vi "RT Loop - Interlock and Post Mortem Data.vi"(8 "error in (no error)":errorcluster, 9 "Master Configuration":T1, 10 "FPGA Subsystem":refnum<queue>, 11 "Message Handler":refnum<queue>) -> ()   [LabVIEW 2014]
uses:
  support/Message Queue/Message Cluster.ctl
  controls/Master Configuration.ctl
  controls/EPICS Configuration.ctl
  controls/FPGA VI Reference.ctl
  <vilib>/Platform/TimedLoop/XDataNode/timing_clust.ctl
  <vilib>/Platform/TimedLoop/XDataNode/nitl_modes.ctl
  <vilib>/Platform/TimedLoop/XDataNode/wakeup.ctl
  Globals/Global - Monitoring Variables.vi
  <vilib>/rvi/errors/niLvFpgaAdjustHostInterfaceError.vi
  Globals/Global - Configuration Options.vi
  <vilib>/Platform/TimedLoop/XDataNode/XDataNode.xnode
  <vilib>/rvi/interface/nirviReadWriteControl/nirviReadWriteControl.xnode
  <vilib>/rvi/interface/nirviMethod/nirviMethod.xnode
  support/Message Queue/Message Queue.lvlib
  <vilib>/FPGAPlugInAG/Dynamic/niLvFpga_ReadFifo_Dynamic.vi
  <vilib>/rvi/errors/niLvFpgaMergeErrorWithErrorCode.vi
  <vilib>/Platform/TimedLoop/XDataNode/XDNodeRunTimeDep.lvlib
  <vilib>/rvi/interface/Simulation/niFpgaSimulationCallBeginRW.vi
  NiFpgaLv.dll
  <vilib>/FPGAPlugInAG/Dynamic/niLvFpga_StopFifo_Dynamic.vi
panel:
  in  "stop":bool
  out "Finished Late?":bool
  out "Iteration Duration":i64
  out "error out 2":errorcluster
  out "error out":errorcluster
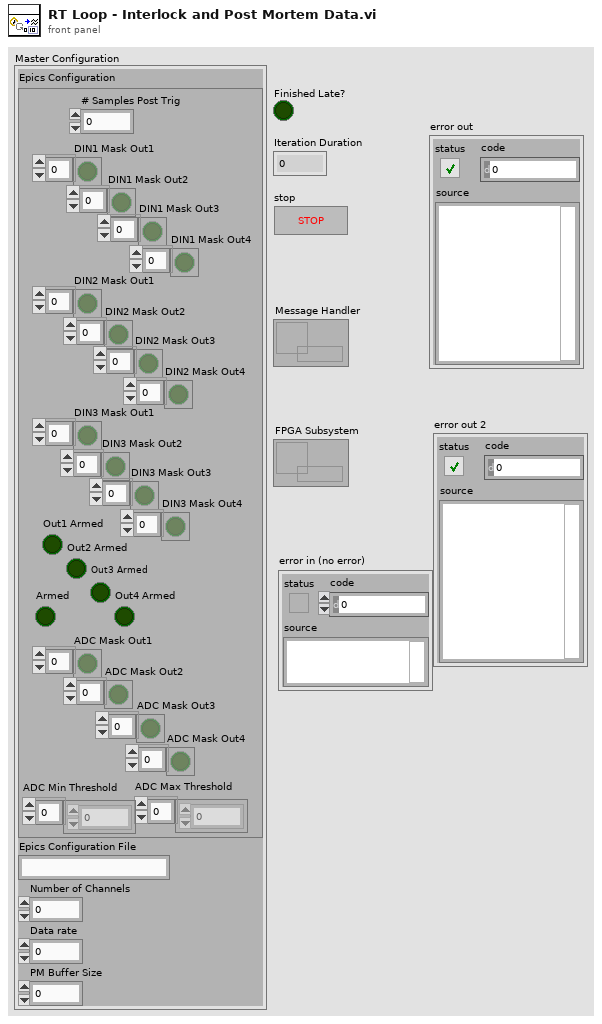
[diagram p1: front panel]
types:
  T1 = typedef "Master Configuration.ctl" = cluster{"Epics Configuration":T2, "Epics Configuration File":string, "Number of Channels":u8, "Data rate":u32, "PM Buffer Size":u32}
  T2 = typedef "EPICS Configuration.ctl" = cluster{"DIN1 Mask Out1":bool[], "# Samples Post Trig":u32, "Armed":bool, "ADC Mask Out1":bool[], "ADC Max Threshold":dbl[], "ADC Min Threshold":dbl[], "DIN1 Mask Out2":bool[], "DIN1 Mask Out3":bool[], "DIN1 Mask Out4":bool[], "Out3 Armed":bool, "Out1 Armed":bool, "Out4 Armed":bool, "Out2 Armed":bool, "DIN2 Mask Out1":bool[], "DIN2 Mask Out2":bool[], "DIN2 Mask Out3":bool[], "DIN2 Mask Out4":bool[], "DIN3 Mask Out1":bool[], "DIN3 Mask Out2":bool[], "DIN3 Mask Out3":bool[], "DIN3 Mask Out4":bool[], "ADC Mask Out2":bool[], "ADC Mask Out3":bool[], "ADC Mask Out4":bool[]}
  T3 = typedef "FPGA VI Reference.ctl" = refnum<k20>
  T4 = typedef "XDNodeRunTimeDep.lvlib/timing_clust.ctl" = cluster{"Expected End [f-1]":u64, "Actual End [f-1]":u64, "Finished Late? [f-1]":bool, "Expected End [i-1]":u64, "Actual End [i-1]":u64, "Finished Late? [i-1]":bool, "Expected Start [i]":u64, "Actual Start [i]":u64, "Expected Start [f]":u64, "Actual Start [f]":u64, "Source Name":string, "Structure Name":string, "Period":i64, "Deadline":i64, "Offset":i64, "Start":i64, "Priority":i32, "Timeout":i32, "Mode":T5, "Wakeup Reason":T6, "Error":errorcluster, "Source Type":string, "Secondary Source Type":string, "Global End Time":u64, "Global Start Time":u64, "Frame Duration":u64, "Iteration Duration":u64, "Assigned CPU":i32, "I/O Scan Engine Mode":u32}
  T5 = typedef "XDNodeRunTimeDep.lvlib/nitl_modes.ctl" = enum32{"No Change", "Process missed periods, maintain original phase", "Discard missed periods, maintain original phase", "Process missed periods, ignore original phase", "Discard missed periods, ignore original phase"}
  T6 = typedef "XDNodeRunTimeDep.lvlib/wakeup.ctl" = enum32{"Normal", "Aborted", "Asynchronous wakeup", "Timing source error", "Timed loop error", "Timeout"}
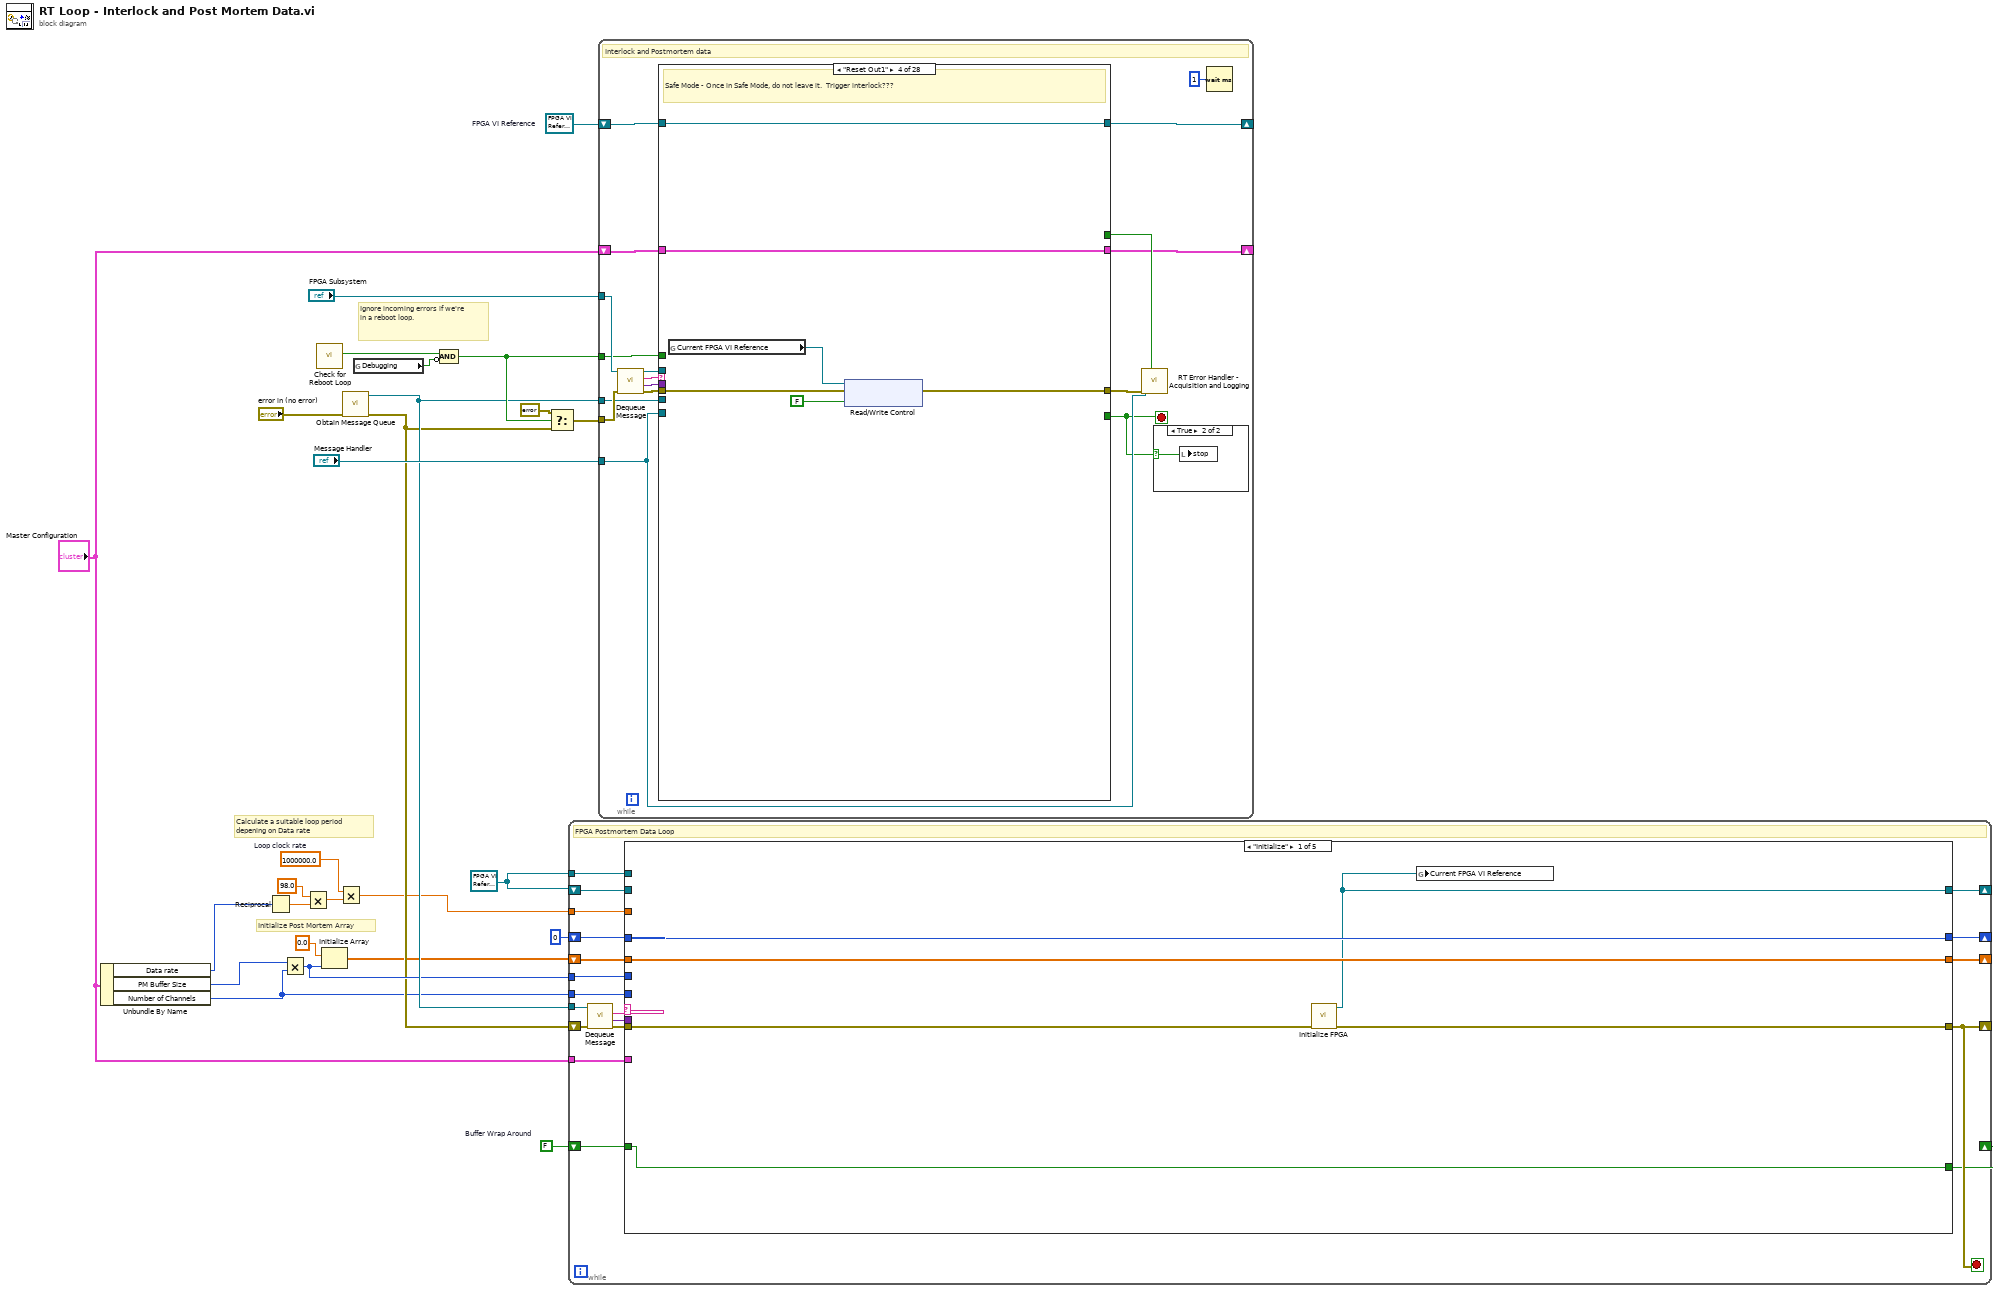
[diagram p0: block diagram]
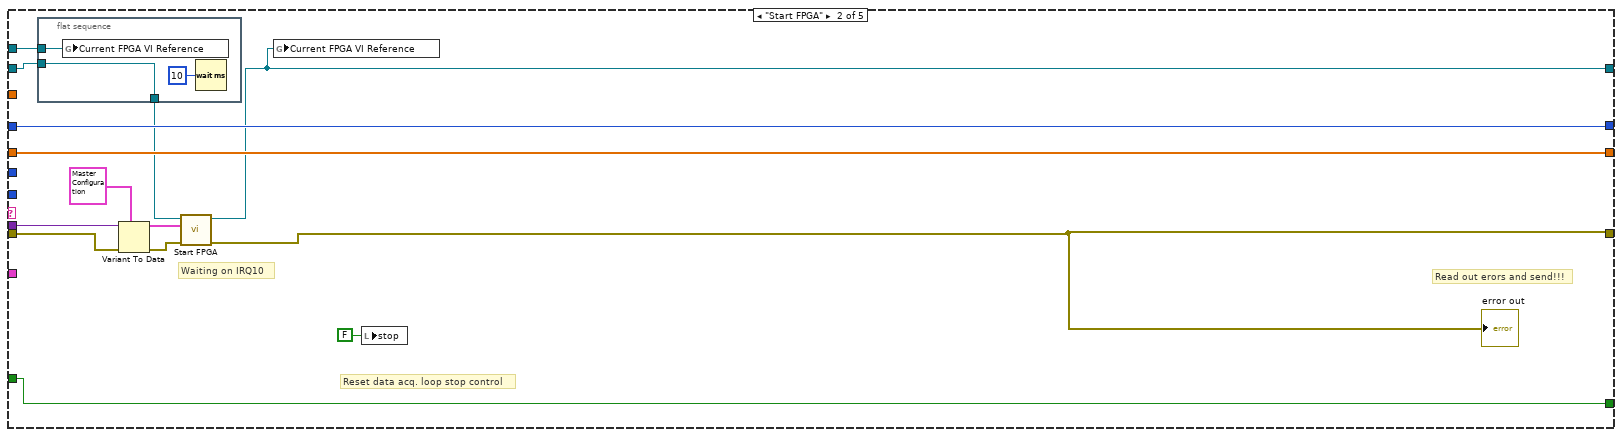
[diagram p2: hidden frame]
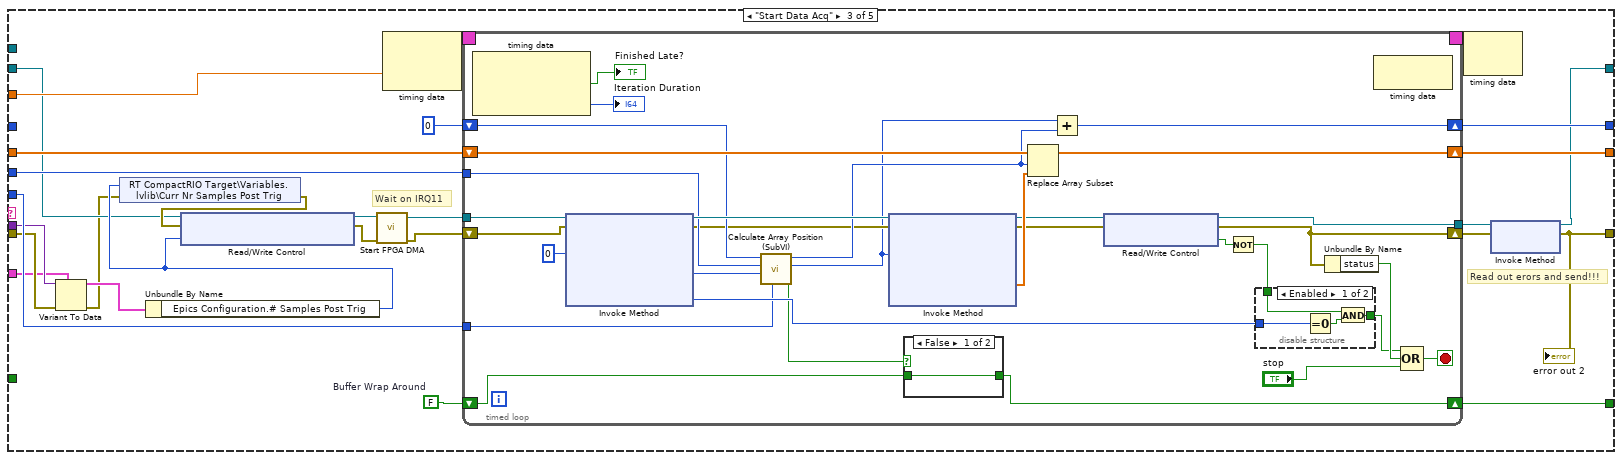
[diagram p3: hidden frame]
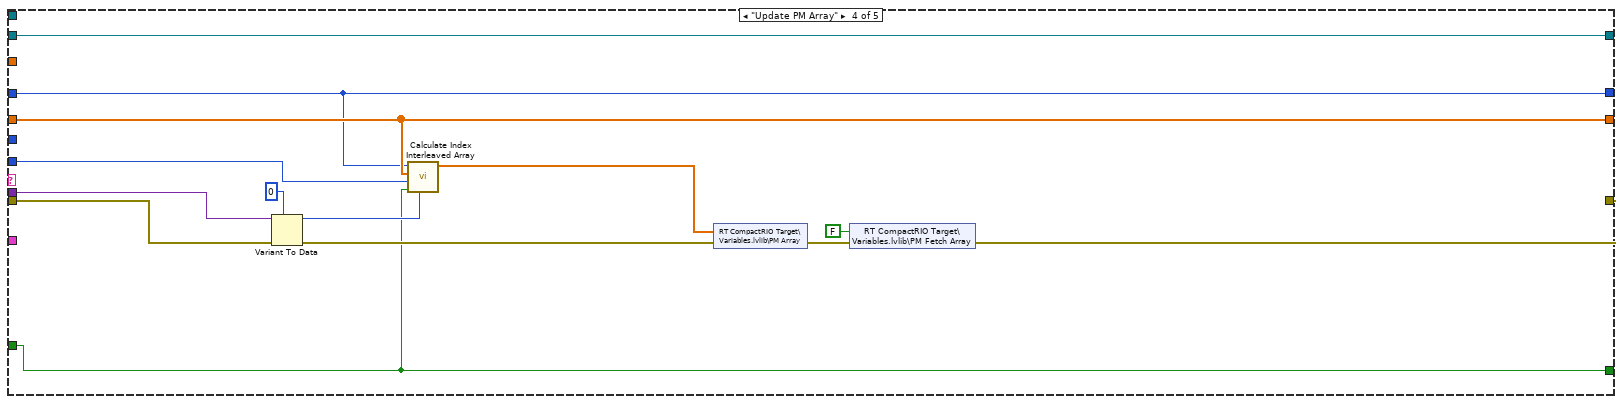
[diagram p6: hidden frame]
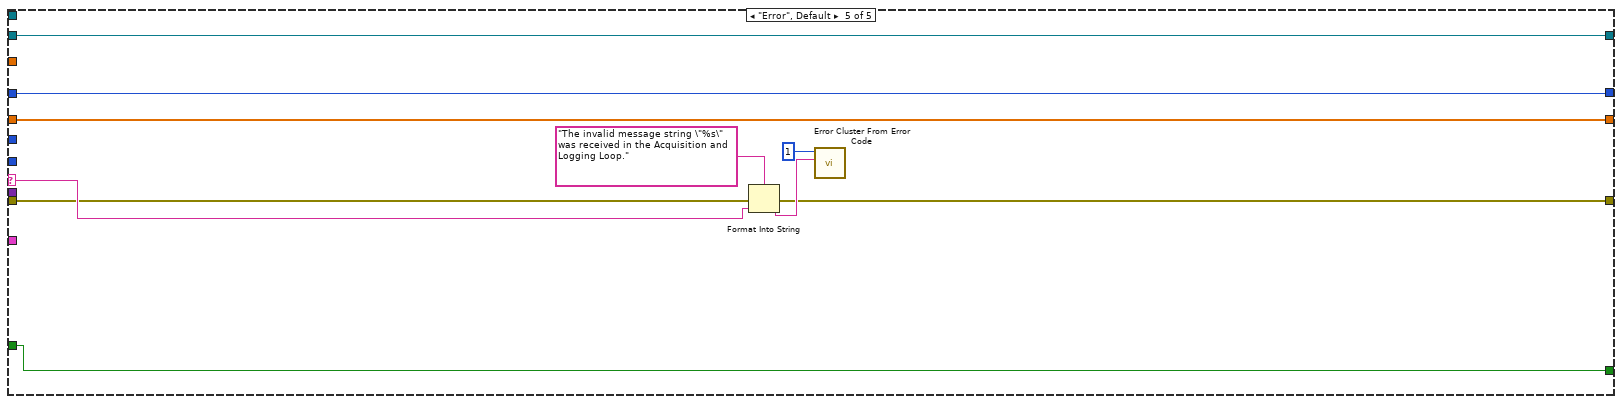
[diagram p7: hidden frame]
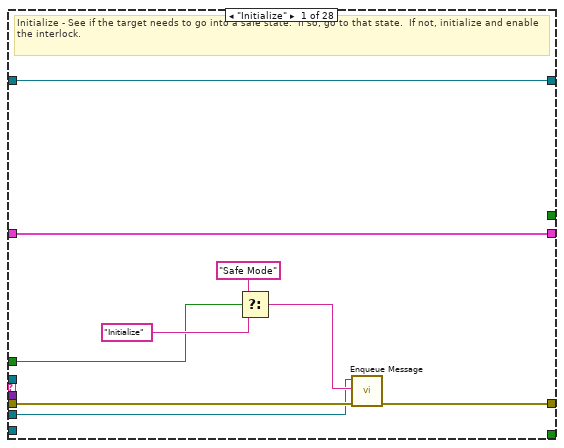
[diagram p9: hidden frame]
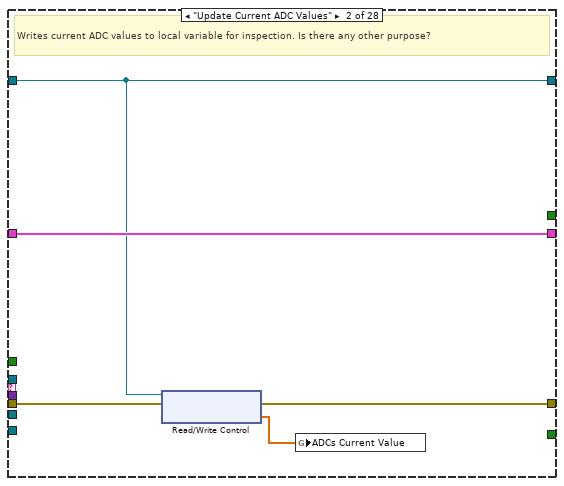
[diagram p10: hidden frame]
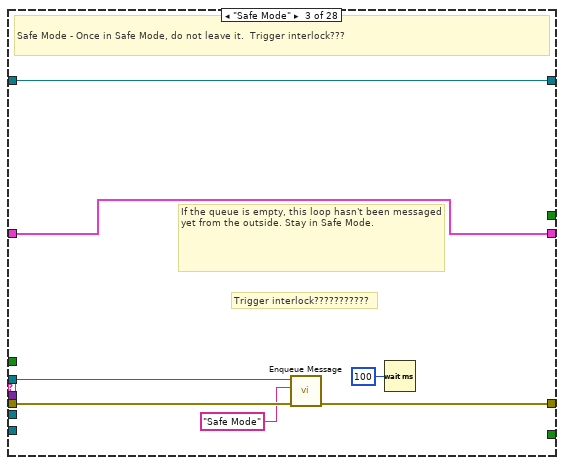
[diagram p11: hidden frame]
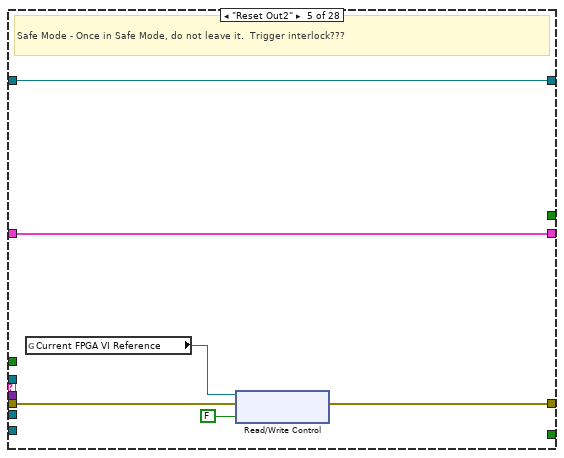
[diagram p12: hidden frame]
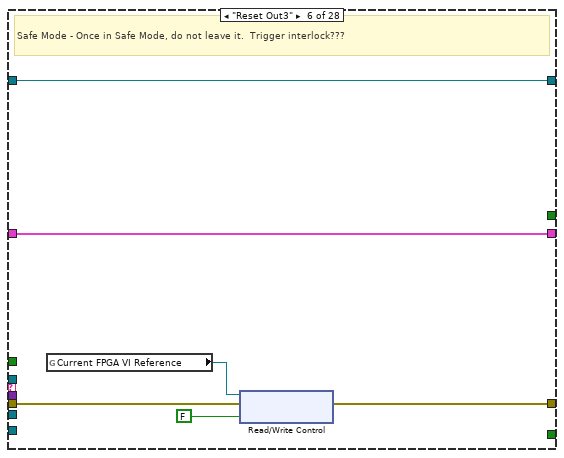
[diagram p13: hidden frame]
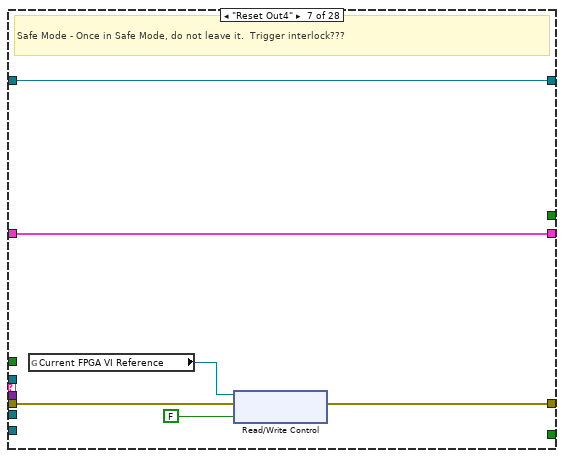
[diagram p14: hidden frame]
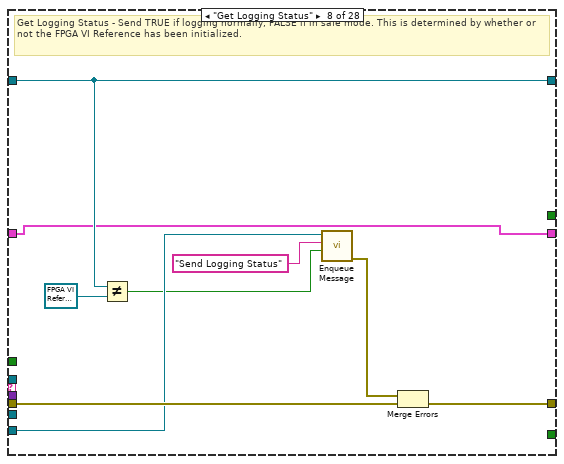
[diagram p15: hidden frame]
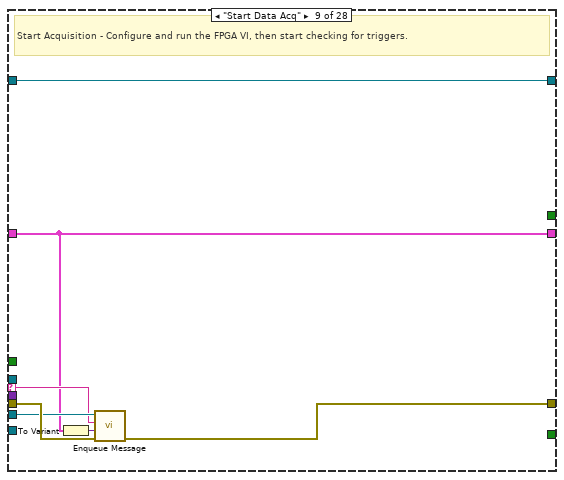
[diagram p16: hidden frame]
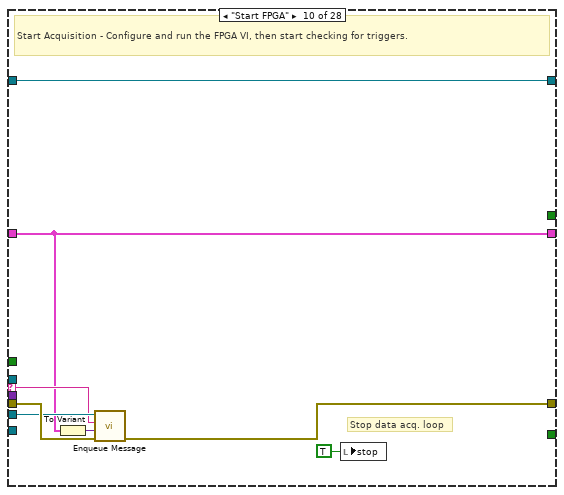
[diagram p17: hidden frame]
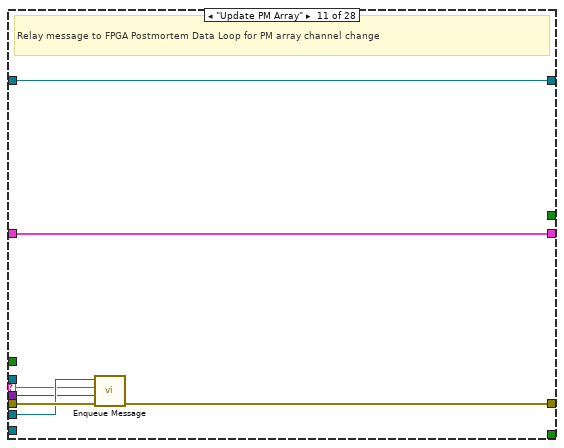
[diagram p18: hidden frame]
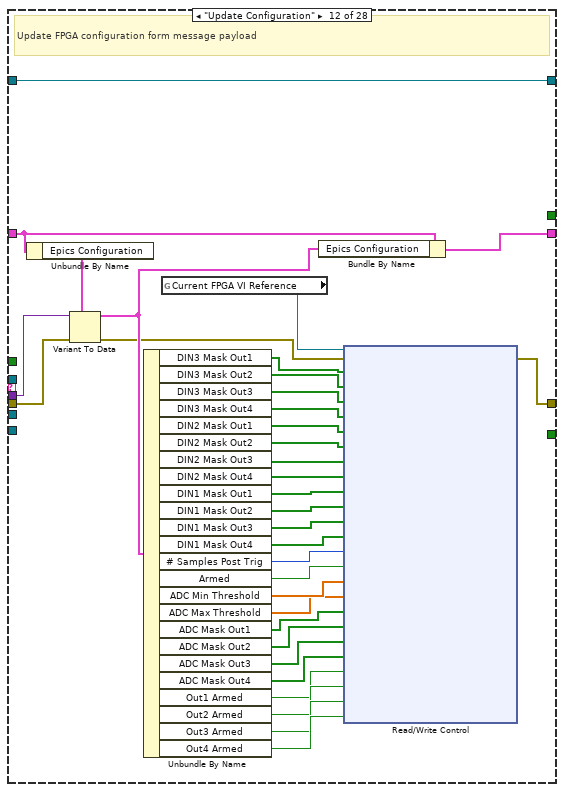
[diagram p19: hidden frame]
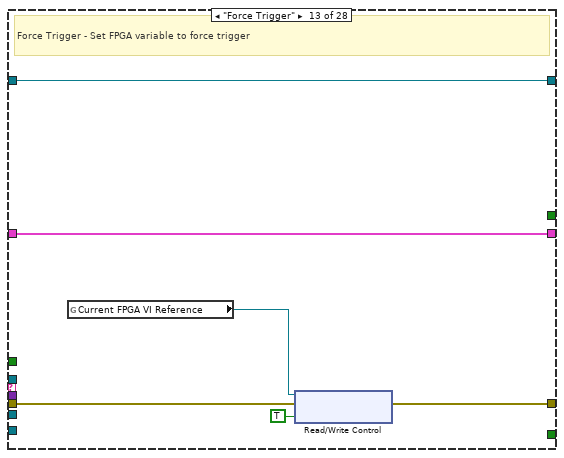
[diagram p20: hidden frame]
diagram:
  w1 = FALSE  # Buffer Wrap Around
  w4 = 1000000.0  # Loop clock rate
  w10 = T3 refnum ("FPGA VI Reference")
  w24 = T3 refnum  # FPGA VI Reference
  # "Calculate a suitable loop period\ndepening on Data rate"
  # "Initialize Post Mortem Array"
  # "Ignore incoming errors if we're in a reboot loop."
  n1 = Unbundle By Name("Master Configuration") -> ("Data rate"=w8:u32, "PM Buffer Size"=w9:u32, "Number of Channels"=w11:u8)
  n2 = Reciprocal(x=w8) -> (1/x=w7:dbl)
  n3 = Multiply(x=w9, y=w11) -> (x*y=w16:u32)
  n4 = Multiply(x=98.0, y=w7) -> (x*y=w5:dbl)
  n5 = call "Check for Reboot Loop.vi"() -> ("Start in Safe Mode?"=w21:bool)  [unwired: 10 in, 1 out]
  n6 = Initialize Array(sgl 0.0, w16) -> (w13:sgl[])
  n7 = Multiply(x=w4, y=w5) -> (x*y=w3:dbl)
  n8 = call "Obtain Message Queue.vi"("error in (no error)"="error in (no error)") -> ("error out"=w14:errorcluster, "Message Queue"=w17:refnum<queue>)  [unwired: 9 in]
  n9 = global read "Global - Configuration Options.vi" "Debugging"() -> (w20:bool)
  n10 = Compound Arithmetic op=AND(w21, invert w20) -> (w19:bool)
  n11 = Select(t=errorcluster {"status"=FALSE, "code"=0, "source"=""}, s=w19, f=w14) -> (s? t:f=w23:errorcluster)
  n12 = while {
    tunnel: w17 -> [w40]
    shift-right: [w43] -> _
    shift-left: w14 -> [w45]
    tunnel: w16 -> [w44]
    shift-right: [w41] -> _
    shift-left: w13 -> [w42]
    shift-right: [w36] -> _
    shift-left: u32 0 ("y") -> [w35]
    tunnel: w11 -> [w34]
    shift-right: [w32] -> _
    shift-left: w10 -> [w33]
    tunnel: w10 -> [w31]
    tunnel: w3 -> [w30]
    tunnel: "Master Configuration" -> [w29]
    shift-right: [w27] -> _
    shift-left: w1 -> [w28]
    stop <- w43 stop-if-true
    # "FPGA Postmortem Data Loop"
    n13 = call "Dequeue Message.vi"("error in (no error)"=w45, "Message Queue"=w40) -> ("error out"=w37:errorcluster, "Message Data"=w38:variant, "Message"=w39:string)  [unwired: 6 in, 1 out]
    n14 = case shown="\"Initialize\"" w39 {
      selector: w39 -> [_ _ _ _ w160]
      tunnel: [w48 w52 w87 w144 w158] -> w43
      tunnel: w44 -> [_ _ w92 _ _]
      tunnel: w42 -> [w51 w65 w91 w150 w164]
      tunnel: [w51 w65 w90 w150 w164] -> w41
      tunnel: w38 -> [_ w64 w82 w154 _]
      tunnel: w37 -> [w49 w63 w81 w153 w159]
      tunnel: [w50 w60 w89 w149 w157] -> w36
      tunnel: w35 -> [w50 w60 _ w149 w157]
      tunnel: w34 -> [_ _ w84 w148 _]
      tunnel: [w47 w56 w85 w142 w156] -> w32
      tunnel: w33 -> [_ w54 w76 w142 w156]
      tunnel: w31 -> [_ w57 _ _ _]
      tunnel: w30 -> [_ _ w83 _ _]
      tunnel: w29 -> [_ _ w80 _ _]
      tunnel: w28 -> [w46 w53 _ w141 w155]
      tunnel: [w46 w53 w69 w141 w155] -> w27
      frame "Initialize" {
        n15 = call "Initialize FPGA.vi"("error in (no error)"=w49) -> ("error out"=w48:errorcluster, "FPGA VI Reference"=w47:T3)  [unwired: 9 in]
        n16 = global write "Global - Monitoring Variables.vi" "Current FPGA VI Reference"(w47) -> ()
      }
      frame "Start FPGA" {
        # "Waiting on IRQ10"
        # "Reset data acq. loop stop control"
        # "Read out erors and send!!!"
        n17 = flat-sequence {
          tunnel: w57 -> [w68]
          tunnel: [w67] -> w55
          tunnel: w54 -> [w67]
          frame #0 {
            n18 = global write "Global - Monitoring Variables.vi" "Current FPGA VI Reference"(w68) -> ()
            n19 = Wait (ms)(milliseconds to wait=u32 10) -> ()  [unwired: 1 out]
          }
        }
        n20 = Variant To Data(error in=w63, type=T1 {"Epics Configuration"={"DIN1 Mask Out1"=[], "# Samples Post Trig"=5, "Armed"=FALSE, "ADC Mask Out1"=[], "ADC Max Threshold"=[], "ADC Min Threshold"=[], "DIN1 Mask Out2"=[], "DIN1 Mask Out3"=[], "DIN1 Mask Out4"=[], "Out3 Armed"=FALSE, "Out1 Armed"=FALSE, "Out4 Armed"=FALSE, "Out2 Armed"=FALSE, "DIN2 Mask Out1"=[], "DIN2 Mask Out2"=[], "DIN2 Mask Out3"=[], "DIN2 Mask Out4"=[], "DIN3 Mask Out1"=[], "DIN3 Mask Out2"=[], "DIN3 Mask Out3"=[], "DIN3 Mask Out4"=[], "ADC Mask Out2"=[], "ADC Mask Out3"=[], "ADC Mask Out4"=[]}, "Epics Configuration File"="/EpicsConfig.cfg", "Number of Channels"=0, "Data rate"=0, "PM Buffer Size"=0} ("Acquisition and Logging Configuration"), Variant=w64) -> (data=w59:T1, error out=w62:errorcluster)
        n21 = call "Start FPGA.vi"("error in (no error)"=w62, "Master Configuration"=w59, "FPGA VI Reference"=w55) -> ("error out"=w52:errorcluster, "FPGA VI Reference"=w56:T3)  [unwired: 7 in]
        "error out" <- w52
        n22 = global write "Global - Monitoring Variables.vi" "Current FPGA VI Reference"(w56) -> ()
        n23 = local write "stop"(FALSE ("stop")) -> ()
      }
      frame "Start Data Acq" {
        w70 = FALSE  # Buffer Wrap Around
        # "Wait on IRQ11"
        # "Read out erors and send!!!"
        n24 = Variant To Data(error in=w81, type=w80, Variant=w82) -> (data=w79:T1, error out=w75:errorcluster)
        n25 = Unbundle By Name(w79) -> ("Epics Configuration.# Samples Post Trig"=w77:u32)
        n26 = shared-variable "RT CompactRIO Target\\Variables.lvlib\\Curr Nr Samples Post Trig"(w77, error in=w75) -> (error out=w78:errorcluster)
        n27 = xnode "Read/Write Control"("FPGA VI Reference In"=w76, "error in"=w78, "Number samples after trigger"=w77) -> ("FPGA VI Reference Out"=w74:T3, "error out"=w73:errorcluster)
        n28 = call "Start FPGA DMA.vi"("error in (no error)"=w73, "FPGA VI Reference"=w74) -> ("error out"=w72:errorcluster, "FPGA VI Reference"=w71:T3)  [unwired: 7 in, 1 out]
        n29 = node-c288(w83) -> (w95:T4)  [unwired: 1 in]
        n30 = timed-loop {
          tunnel: w71 -> [w116]
          shift-right: [w124] -> w90
          shift-left: w91 -> [w125]
          tunnel: w92 -> [w108]
          timing: w95 -> [_]
          timing-out: [_] -> w94
          shift-right: [w103] -> w89
          shift-left: u32 0 ("y") -> [w106]
          shift-right: [w112] -> w88
          shift-left: w72 -> [w117]
          tunnel: [w101] -> w86
          tunnel: w84 -> [w99]
          shift-right: [w96] -> w69
          shift-left: w70 -> [w97]
          stop <- w105 stop-if-true
          n31 = node-c288() -> (→"Finished Late?":bool, →"Iteration Duration":i64)  [unwired: 1 in, 1 out]
          n32 = xnode "Invoke Method"("FPGA VI Reference In"=w116, "error in"=w117, "Number of Elements"=u32 0) -> ("FPGA VI Reference Out"=w115:T3, "error out"=w104:errorcluster, "Elements Remaining"=w109:u32)  [unwired: 1 in, 1 out]
          n33 = call "Calculate Array Position (SubVI).vi"("Number of Channels"=w99, "Elements Remaining"=w109, "FIFO Size"=w108, "Position"=w106) -> ("Buffer Wrap Around"=w98:bool, "Elements to read"=w102:u32, "New Position"=w107:u32)  [unwired: 5 in]
          n34 = xnode "Invoke Method"("FPGA VI Reference In"=w115, "error in"=w104, "Number of Elements"=w102) -> ("FPGA VI Reference Out"=w114:T3, "error out"=w113:errorcluster, "Data"=w123:sgl[])  [unwired: 1 in, 1 out]
          n35 = case shown="False" w98 {
            selector: w98 -> [_ w127]
            tunnel: w97 -> [w126 _]
            tunnel: [w126 w127] -> w96
            frame False {
            }
            frame True {
            }
          }
          n36 = Replace Array Subset(array=w125, new element=w123, index=w107) -> (w124:sgl[])
          n37 = Add(x=w102, y=w107) -> (x+y=w103:u32)
          n38 = xnode "Read/Write Control"("FPGA VI Reference In"=w114, "error in"=w113) -> ("FPGA VI Reference Out"=w101:T3, "error out"=w112:errorcluster, "Data Acq Running"=w111:bool)
          n39 = Not(x=w111) -> (.not. x?=w100:bool)
          n40 = disable-structure shown="Enabled" {
            disable-tunnel: w100 -> [w131 w132]
            disable-tunnel: [w130 w132] -> w110
            disable-tunnel: w109 -> [w128 _]
            frame Enabled {
              n41 = Equal To 0?(x=w128) -> (x = 0?=w129:bool)
              n42 = And(x=w131, y=w129) -> (x .and. y?=w130:bool)
            }
            frame Disabled {
            }
          }
          n43 = Unbundle By Name(w112) -> ("status"=w122:bool)
          n44 = node-c288() -> ()  [unwired: 1 in, 1 out]
          n45 = Compound Arithmetic op=OR(w110, w122, "stop") -> (w105:bool)
        }
        n46 = node-c288(w94) -> ()  [unwired: 1 out]
        n47 = xnode "Invoke Method"("FPGA VI Reference In"=w86, "error in"=w88) -> ("FPGA VI Reference Out"=w85:T3, "error out"=w87:errorcluster)
        "error out 2" <- w87
      }
      frame "Update PM Array" {
        n48 = Variant To Data(error in=w153, type=0, Variant=w154) -> (data=w151:i32, error out=w146:errorcluster)
        n49 = call "Calculate Index Interleaved Array.vi"("Index"=w151, "Buffer Wrap Around"=w141, "Number of Channels"=w148, "Interleaved Array"=w150, "Position Zero"=w149) -> ("Array"=w147:sgl[])  [unwired: 6 in]
        n50 = shared-variable "RT CompactRIO Target\\Variables.lvlib\\PM Array"(w147, error in=w146) -> (error out=w145:errorcluster)
        n51 = shared-variable "RT CompactRIO Target\\Variables.lvlib\\PM Fetch Array"(FALSE ("Fetch PM Array"), error in=w145) -> (error out=w144:errorcluster)
      }
      frame "Error", Default {
        n52 = Format Into String(format string="The invalid message string \"%s\" was received in the Acquisition and Logging Loop." ("Unknown Message Error Text"), error in=w159, w160) -> (resulting string=w161:string, error out=w158:errorcluster)  [unwired: 1 in]
        n53 = call <vilib>:"Error Cluster From Error Code.vi"("error message (\"\")"=w161, "error code (0)"=1) -> ()  [unwired: 7 in, 1 out]
      }
    }
  }
  n54 = while {
    tunnel: "FPGA Subsystem" -> [w178]
    tunnel: "Message Handler" -> [w171]
    shift-right: [w174] -> _
    shift-left: w24 -> [w175]
    tunnel: w23 -> [w169]
    tunnel: w19 -> [w168]
    tunnel: w17 -> [w167]
    shift-right: [w166] -> _
    shift-left: "Master Configuration" -> [w173]
    stop <- w165 stop-if-true
    # "Interlock and Postmortem data"
    n55 = call "Dequeue Message.vi"("error in (no error)"=w169, "Message Queue"=w178) -> ("error out"=w181:errorcluster, "Message Data"=w179:variant, "Message"=w180:string, "dup Message Queue"=w176:refnum<queue>)  [unwired: 6 in]
    n56 = case "Message Cases" shown="\"Reset Out1\"" w180 {
      selector: w180 -> [_ _ _ _ _ _ _ _ w239 w247 w254 _ _ _ _ _ _ _ _ _ _ _ _ _ _ _ _ w404]
      tunnel: w176 -> [_ _ w201 _ _ _ _ _ _ _ _ _ _ _ _ _ _ _ _ _ _ _ _ _ w387 _ _ _]
      tunnel: w181 -> [w190 w194 w202 w205 w211 w217 w223 w236 w243 w251 w258 w291 w296 w302 w308 w314 w320 w326 w332 w341 w350 w359 w368 w374 w383 w391 w394 _]
      tunnel: [w186 w193 w200 w204 w210 w216 w222 w233 w242 w250 w257 w284 w295 w301 w307 w313 w319 w325 w331 w335 w345 w354 w363 w373 w384 w390 w398 w402] -> w177
      tunnel: [_ _ _ _ _ _ _ _ _ _ _ _ _ _ _ _ _ _ _ _ _ _ _ _ TRUE _ _ _] -> w165
      tunnel: w179 -> [_ _ _ _ _ _ _ _ _ _ w253 w290 _ _ _ _ _ _ _ _ _ _ _ _ _ _ w396 _]
      tunnel: w175 -> [w191 w195 w203 w209 w215 w221 w227 w235 w241 w249 w256 w292 w298 w304 w310 w316 w322 w328 w334 w343 w352 w361 w370 w376 w380 w389 w397 w400]
      tunnel: [w191 w195 w203 w209 w215 w221 w227 w235 w241 w249 w256 w292 w298 w304 w310 w316 w322 w328 w334 w343 w352 w361 w370 w376 w380 w389 w397 w400] -> w174
      tunnel: w173 -> [w184 w196 w197 w208 w214 w220 w226 w228 w238 w245 w252 w288 w297 w303 w309 w315 w321 w327 w333 w342 w351 w360 w369 w375 w379 w388 w395 w399]
      tunnel: w171 -> [_ _ _ _ _ _ _ w234 _ _ _ _ _ _ _ _ _ _ _ w336 w344 w353 w362 _ _ _ _ _]
      tunnel: [_ _ _ _ _ _ _ _ _ _ _ _ _ _ _ _ _ _ _ _ _ _ _ _ w381 _ _ _] -> w170
      tunnel: w168 -> [w185 _ _ _ _ _ _ _ _ _ _ _ _ _ _ _ _ _ _ _ _ _ _ _ _ _ _ _]
      tunnel: w167 -> [w183 _ _ _ _ _ _ _ w240 w248 w255 _ _ _ _ _ _ _ _ _ _ _ _ _ w377 _ _ _]
      tunnel: [w184 w196 w197 w208 w214 w220 w226 w228 w238 w245 w252 w287 w297 w303 w309 w315 w321 w327 w333 w342 w351 w360 w369 w375 w379 w388 w392 w399] -> w166
      frame "Initialize" {
        # "Initialize - See if the target needs to go into a safe state.  If so, go to that state.  If not, initialize and enable the interlock."
        n57 = Select(t="Safe Mode", s=w185, f="Initialize") -> (s? t:f=w187:string)
        n58 = call "Enqueue Message.vi"("error in (no error)"=w190, "Message"=w187, "Message Queue"=w183) -> ("error out"=w186:errorcluster)  [unwired: 7 in, 1 out]
      }
      frame "Update Current ADC Values" {
        # "Writes current ADC values to local variable for inspection. Is there any other purpose?"
        n59 = xnode "Read/Write Control"("FPGA VI Reference In"=w195, "error in"=w194) -> ("error out"=w193:errorcluster, "Current sample"=w192:sgl[])  [unwired: 1 out]
        n60 = global write "Global - Monitoring Variables.vi" "ADCs Current Value"(w192) -> ()
      }
      frame "Safe Mode" {
        # "Trigger interlock???????????"
        # "If the queue is empty, this loop hasn't been messaged yet from the outside. Stay in Safe Mode."
        # "Safe Mode - Once in Safe Mode, do not leave it.  Trigger interlock???"
        n61 = call "Enqueue Message.vi"("error in (no error)"=w202, "Message"="Safe Mode", "Message Queue"=w201) -> ("error out"=w200:errorcluster)  [unwired: 7 in, 1 out]
        n62 = Wait (ms)(milliseconds to wait=u32 100) -> ()  [unwired: 1 out]
      }
      frame "Reset Out1" {
        # "Safe Mode - Once in Safe Mode, do not leave it.  Trigger interlock???"
        n63 = global read "Global - Monitoring Variables.vi" "Current FPGA VI Reference"() -> (w206:T3)
        n64 = xnode "Read/Write Control"("FPGA VI Reference In"=w206, "error in"=w205, "Interlock Out1"=FALSE ("External trigger")) -> ("error out"=w204:errorcluster)  [unwired: 1 out]
      }
      frame "Reset Out2" {
        # "Safe Mode - Once in Safe Mode, do not leave it.  Trigger interlock???"
        n65 = global read "Global - Monitoring Variables.vi" "Current FPGA VI Reference"() -> (w212:T3)
        n66 = xnode "Read/Write Control"("FPGA VI Reference In"=w212, "error in"=w211, "Interlock Out2"=FALSE ("External trigger")) -> ("error out"=w210:errorcluster)  [unwired: 1 out]
      }
      frame "Reset Out3" {
        # "Safe Mode - Once in Safe Mode, do not leave it.  Trigger interlock???"
        n67 = global read "Global - Monitoring Variables.vi" "Current FPGA VI Reference"() -> (w218:T3)
        n68 = xnode "Read/Write Control"("FPGA VI Reference In"=w218, "error in"=w217, "Interlock Out3"=FALSE ("External trigger")) -> ("error out"=w216:errorcluster)  [unwired: 1 out]
      }
      frame "Reset Out4" {
        # "Safe Mode - Once in Safe Mode, do not leave it.  Trigger interlock???"
        n69 = global read "Global - Monitoring Variables.vi" "Current FPGA VI Reference"() -> (w224:T3)
        n70 = xnode "Read/Write Control"("FPGA VI Reference In"=w224, "error in"=w223, "Interlock Out4"=FALSE ("External trigger")) -> ("error out"=w222:errorcluster)  [unwired: 1 out]
      }
      frame "Get Logging Status" {
        # "Get Logging Status - Send TRUE if logging normally, FALSE if in safe mode. This is determined by whether or not the FPGA VI Reference has been initialized."
        n71 = Not Equal?(x=w235, y=T3 refnum ("FPGA VI Reference")) -> (x != y?=w231:bool)
        n72 = call "Enqueue Message.vi"("Message Data"=w231, "Message"="Send Logging Status", "Message Queue"=w234) -> ("error out"=w232:errorcluster)  [unwired: 7 in, 1 out]
        n73 = Merge Errors(w232, w236) -> (w233:errorcluster)
      }
      frame "Start Data Acq" {
        # "Start Acquisition - Configure and run the FPGA VI, then start checking for triggers."
        n74 = To Variant(anything=w238) -> (Variant=w237:variant)
        n75 = call "Enqueue Message.vi"("error in (no error)"=w243, "Message Data"=w237, "Message"=w239, "Message Queue"=w240) -> ("error out"=w242:errorcluster)  [unwired: 6 in, 1 out]
      }
      frame "Start FPGA" {
        # "Stop data acq. loop"
        # "Start Acquisition - Configure and run the FPGA VI, then start checking for triggers."
        n76 = To Variant(anything=w245) -> (Variant=w246:variant)
        n77 = call "Enqueue Message.vi"("error in (no error)"=w251, "Message Data"=w246, "Message"=w247, "Message Queue"=w248) -> ("error out"=w250:errorcluster)  [unwired: 6 in, 1 out]
        n78 = local write "stop"(TRUE ("stop")) -> ()
      }
      frame "Update PM Array" {
        # "Relay message to FPGA Postmortem Data Loop for PM array channel change"
        n79 = call "Enqueue Message.vi"("error in (no error)"=w258, "Message Data"=w253, "Message"=w254, "Message Queue"=w255) -> ("error out"=w257:errorcluster)  [unwired: 6 in, 1 out]
      }
      frame "Update Configuration" {
        # "Update FPGA configuration form message payload"
        n80 = Unbundle By Name(w288) -> ("Epics Configuration"=w289:T2)
        n81 = Variant To Data(error in=w291, type=w289, Variant=w290) -> (data=w286:T2, error out=w285:errorcluster)
        n82 = Unbundle By Name(w286) -> ("DIN3 Mask Out1"=w263:bool[], "DIN3 Mask Out2"=w264:bool[], "DIN3 Mask Out3"=w265:bool[], "DIN3 Mask Out4"=w266:bool[], "DIN2 Mask Out1"=w267:bool[], "DIN2 Mask Out2"=w268:bool[], "DIN2 Mask Out3"=w269:bool[], "DIN2 Mask Out4"=w270:bool[], "DIN1 Mask Out1"=w278:bool[], "DIN1 Mask Out2"=w277:bool[], "DIN1 Mask Out3"=w276:bool[], "DIN1 Mask Out4"=w275:bool[], "# Samples Post Trig"=w283:u32, "Armed"=w281:bool, "ADC Min Threshold"=w280:dbl[], "ADC Max Threshold"=w279:dbl[], "ADC Mask Out1"=w259:bool[], "ADC Mask Out2"=w260:bool[], "ADC Mask Out3"=w261:bool[], "ADC Mask Out4"=w262:bool[], "Out1 Armed"=w271:bool, "Out2 Armed"=w272:bool, "Out3 Armed"=w273:bool, "Out4 Armed"=w274:bool)
        n83 = global read "Global - Monitoring Variables.vi" "Current FPGA VI Reference"() -> (w282:T3)
        n84 = Bundle By Name(cluster=w288, "Epics Configuration"=w286) -> (w287:T1)
        n85 = xnode "Read/Write Control"("FPGA VI Reference In"=w282, "error in"=w285, "DIN3 Mask Out1"=w263, "DIN3 Mask Out2"=w264, "DIN3 Mask Out3"=w265, "DIN3 Mask Out4"=w266, "DIN2 Mask Out1"=w267, "DIN2 Mask Out2"=w268, "DIN2 Mask Out3"=w269, "DIN2 Mask Out4"=w270, "DIN1 Mask Out1"=w278, "DIN1 Mask Out2"=w277, "DIN1 Mask Out3"=w276, "DIN1 Mask Out4"=w275, "Number samples after trigger"=w283, "Interlock on"=w281, "ADC Threshold min value"=w280, "ADC Threshold max value"=w279, "ADC Mask Out1"=w259, "ADC Mask Out2"=w260, "ADC Mask Out3"=w261, "ADC Mask Out4"=w262, "Out1 Armed"=w271, "Out2 Armed"=w272, "Out3 Armed"=w273, "Out4 Armed"=w274) -> ("error out"=w284:errorcluster)  [unwired: 1 out]
      }
      frame "Force Trigger" {
        # "Force Trigger - Set FPGA variable to force trigger"
        n86 = global read "Global - Monitoring Variables.vi" "Current FPGA VI Reference"() -> (w294:T3)
        n87 = xnode "Read/Write Control"("FPGA VI Reference In"=w294, "error in"=w296, "External trigger"=TRUE) -> ("error out"=w295:errorcluster)  [unwired: 1 out]
      }
      frame "Arm" {
        # "Force Trigger - Set FPGA variable to force trigger"
        n88 = global read "Global - Monitoring Variables.vi" "Current FPGA VI Reference"() -> (w300:T3)
        n89 = xnode "Read/Write Control"("FPGA VI Reference In"=w300, "error in"=w302, "Interlock on"=TRUE ("External trigger")) -> ("error out"=w301:errorcluster)  [unwired: 1 out]
      }
      frame "Out1 Arm" {
        # "Force Trigger - Set FPGA variable to force trigger"
        n90 = global read "Global - Monitoring Variables.vi" "Current FPGA VI Reference"() -> (w306:T3)
        n91 = xnode "Read/Write Control"("FPGA VI Reference In"=w306, "error in"=w308, "Out1 Armed"=TRUE ("External trigger")) -> ("error out"=w307:errorcluster)  [unwired: 1 out]
      }
      frame "Out2 Arm" {
        # "Force Trigger - Set FPGA variable to force trigger"
        n92 = global read "Global - Monitoring Variables.vi" "Current FPGA VI Reference"() -> (w312:T3)
        n93 = xnode "Read/Write Control"("FPGA VI Reference In"=w312, "error in"=w314, "Out2 Armed"=TRUE ("External trigger")) -> ("error out"=w313:errorcluster)  [unwired: 1 out]
      }
      frame "Out3 Arm" {
        # "Force Trigger - Set FPGA variable to force trigger"
        n94 = global read "Global - Monitoring Variables.vi" "Current FPGA VI Reference"() -> (w318:T3)
        n95 = xnode "Read/Write Control"("FPGA VI Reference In"=w318, "error in"=w320, "Out3 Armed"=TRUE ("External trigger")) -> ("error out"=w319:errorcluster)  [unwired: 1 out]
      }
      frame "Out4 Arm" {
        # "Force Trigger - Set FPGA variable to force trigger"
        n96 = global read "Global - Monitoring Variables.vi" "Current FPGA VI Reference"() -> (w324:T3)
        n97 = xnode "Read/Write Control"("FPGA VI Reference In"=w324, "error in"=w326, "Out4 Armed"=TRUE ("External trigger")) -> ("error out"=w325:errorcluster)  [unwired: 1 out]
      }
      frame "Disarm" {
        # "Force Trigger - Set FPGA variable to force trigger"
        n98 = global read "Global - Monitoring Variables.vi" "Current FPGA VI Reference"() -> (w330:T3)
        n99 = xnode "Read/Write Control"("FPGA VI Reference In"=w330, "error in"=w332, "Interlock on"=FALSE ("External trigger")) -> ("error out"=w331:errorcluster)  [unwired: 1 out]
      }
      frame "Out1 Disarm" {
        # "Force Trigger - Set FPGA variable to force trigger"
        n100 = global read "Global - Monitoring Variables.vi" "Current FPGA VI Reference"() -> (w340:T3)
        n101 = xnode "Read/Write Control"("FPGA VI Reference In"=w340, "error in"=w341, "Out1 Armed"=FALSE ("External trigger")) -> ("error out"=w337:errorcluster)  [unwired: 1 out]
        n102 = call "Enqueue Message.vi"("error in (no error)"=w337, "Message"="Clear Rst Out1", "Message Queue"=w336) -> ("error out"=w335:errorcluster)  [unwired: 7 in, 1 out]
      }
      frame "Out2 Disarm" {
        # "Force Trigger - Set FPGA variable to force trigger"
        n103 = global read "Global - Monitoring Variables.vi" "Current FPGA VI Reference"() -> (w349:T3)
        n104 = xnode "Read/Write Control"("FPGA VI Reference In"=w349, "error in"=w350, "Out2 Armed"=FALSE ("External trigger")) -> ("error out"=w346:errorcluster)  [unwired: 1 out]
        n105 = call "Enqueue Message.vi"("error in (no error)"=w346, "Message"="Clear Rst Out2", "Message Queue"=w344) -> ("error out"=w345:errorcluster)  [unwired: 7 in, 1 out]
      }
      frame "Out3 Disarm" {
        # "Force Trigger - Set FPGA variable to force trigger"
        n106 = global read "Global - Monitoring Variables.vi" "Current FPGA VI Reference"() -> (w358:T3)
        n107 = xnode "Read/Write Control"("FPGA VI Reference In"=w358, "error in"=w359, "Out3 Armed"=FALSE ("External trigger")) -> ("error out"=w355:errorcluster)  [unwired: 1 out]
        n108 = call "Enqueue Message.vi"("error in (no error)"=w355, "Message"="Clear Rst Out3", "Message Queue"=w353) -> ("error out"=w354:errorcluster)  [unwired: 7 in, 1 out]
      }
      frame "Out4 Disarm" {
        # "Force Trigger - Set FPGA variable to force trigger"
        n109 = global read "Global - Monitoring Variables.vi" "Current FPGA VI Reference"() -> (w367:T3)
        n110 = xnode "Read/Write Control"("FPGA VI Reference In"=w367, "error in"=w368, "Out4 Armed"=FALSE ("External trigger")) -> ("error out"=w364:errorcluster)  [unwired: 1 out]
        n111 = call "Enqueue Message.vi"("error in (no error)"=w364, "Message"="Clear Rst Out4", "Message Queue"=w362) -> ("error out"=w363:errorcluster)  [unwired: 7 in, 1 out]
      }
      frame "Stop Data Acq" {
        # "Force Trigger - Set FPGA variable to force trigger"
        n112 = global read "Global - Monitoring Variables.vi" "Current FPGA VI Reference"() -> (w372:T3)
        n113 = xnode "Read/Write Control"("FPGA VI Reference In"=w372, "error in"=w374, "Data Acq Stop"=TRUE ("External trigger")) -> ("error out"=w373:errorcluster)  [unwired: 1 out]
      }
      frame "Exit" {
        # "Stop Acquisition and Logging Loop"
        # "Release the message queue reference"
        # "Exit - Close message queues and shut down the FPGA."
        n114 = Release Queue(queue=w387, error in (no error)=w383) -> (error out=w385:errorcluster)  [unwired: 1 in, 2 out]
        n115 = call "FPGA Disarm.vi"("FPGA VI Reference"=w380) -> ("error out"=w382:errorcluster, "Stop FPGA Timeout?"=w381:bool)  [unwired: 9 in]
        n116 = Release Queue(queue=w377, error in (no error)=w385) -> (error out=w378:errorcluster)  [unwired: 1 in, 2 out]
        n117 = Merge Errors(w382, w378) -> (w384:errorcluster)
      }
      frame "---Copy This Frame---" {
        # "Duplicate this frame when creating new messages.  Change this comment in the duplicated frame to describe this message."
        n118 = Merge Errors(w391) -> (w390:errorcluster)
      }
      frame "Update FPGA parameters" {
        # "Update Master Configuration (not currently used)"
        n119 = Variant To Data(error in=w394, type=w395, Variant=w396) -> (data=w392:T1, error out=w393:errorcluster)
        n120 = Merge Errors(w393) -> (w398:errorcluster)
      }
      frame Default {
        # "'Default' case only runs if there is a message that isn't defined in any of the other cases.  Output a programming error."
        n121 = Format Into String(format string="The invalid message string \"%s\" was received in the Acquisition and Logging Loop." ("Unknown Message Error Text"), w404) -> (resulting string=w401:string)  [unwired: 2 in, 1 out]
        n122 = call <vilib>:"Error Cluster From Error Code.vi"("error message (\"\")"=w401, "error code (0)"=1) -> ("error out"=w402:errorcluster)  [unwired: 7 in]
      }
    }
    n123 = call "RT Error Handler - Acquisition and Logging.vi"("Stop FPGA Timeout"=w170, "error in (no error)"=w177, "Message Queue"=w171) -> ()  [unwired: 8 in, 1 out]
    n124 = case shown="True" w165 {
      selector: w165 -> [_ w182]
      frame False {
      }
      frame True {
        n125 = local write "stop"(w182) -> ()
      }
    }
    n126 = Wait (ms)(milliseconds to wait=u32 1) -> ()  [unwired: 1 out]
  }
